vi "CST handler.vi"(0 "System no.":i32=1 min=1 max=4 step=1, 2 "Axis ID's In":string[](array[string]), 3 "Stage names In":string[](array[string]), 5 "error in":errorcluster, 6 "Query SAI? ALL?":bool=TRUE, 7 "Dialog?":bool=TRUE caption="Use dialog to define\nconnected stages?") -> (16 "Axis ID's Out":string[](array[string]), 17 "Stage names Out":string[](array[string]), 19 "error out":errorcluster)   [LabVIEW 2026]
doc: "Defines connected stages for axes, depending on several selections. Requires SAI.vi, SAI?.vi, CST?.vi and ERR?.vi. For Query SAI? ALL? = TRUE, VI determines connected axes by querying SAI? ALL. For Query SAI? = FALSE; Axis ID's IN must contain the correct identifiers of all connected axes. Use dialog to define connected stages? determines if a dialog pops up for the stage selection. If this control is set to FALSE, Stage names In must contain the correct stage names for all connected axes. Empty fields are substituted with \"NOSTAGE\". \n\nC-877, C-884, C-891: Command is available via USB interface only.\nC-867, E-871, E-873: Command is available via USB, USB DaisyChain or RS232 DaisyChain interface only.\nPollux: See HydraPollux_GCS_DLL manual for specialities of the Pollux controller family regarding stage name settings."
panel:
  # "Defines connected stages for axes, depending on several selections. Requires SAI.vi, SAI?.vi, CST?.vi and ERR?.vi."
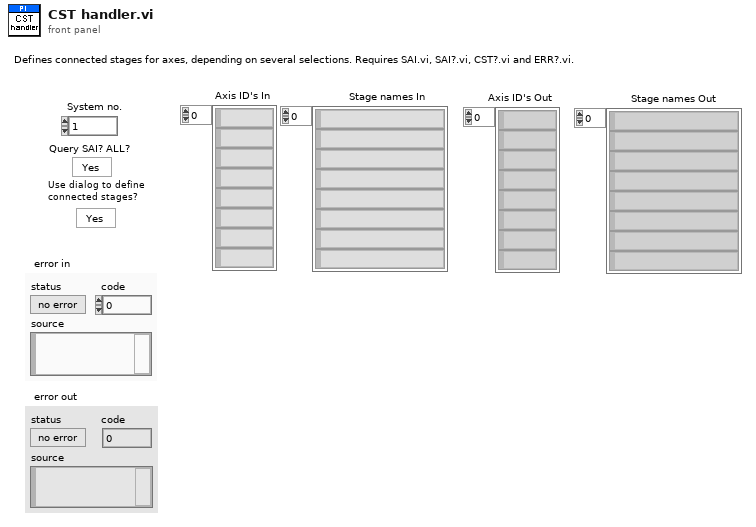
[diagram p1: front panel]
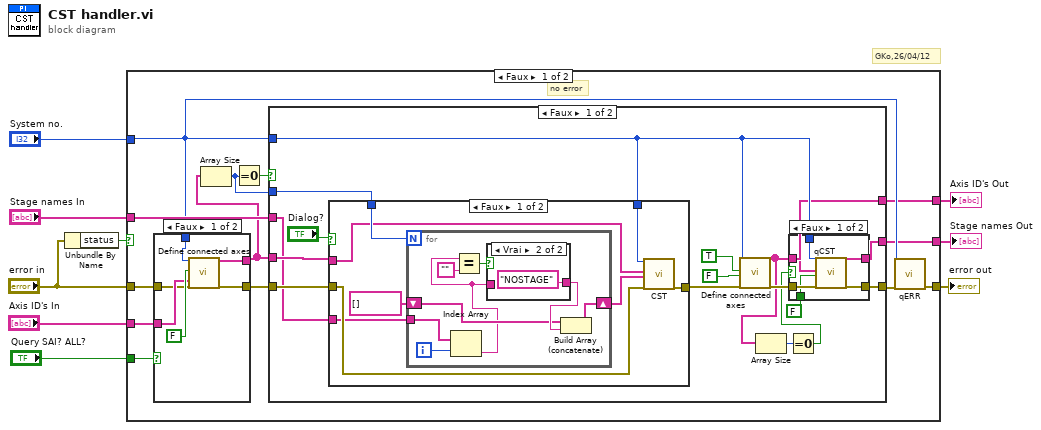
[diagram p0: block diagram]
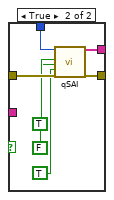
[diagram p2: hidden frame]
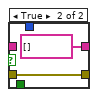
[diagram p3: hidden frame]
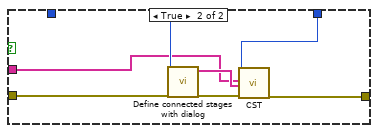
[diagram p5: hidden frame]
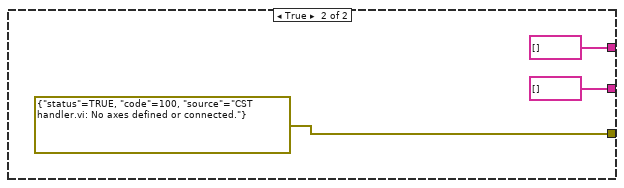
[diagram p6: hidden frame]
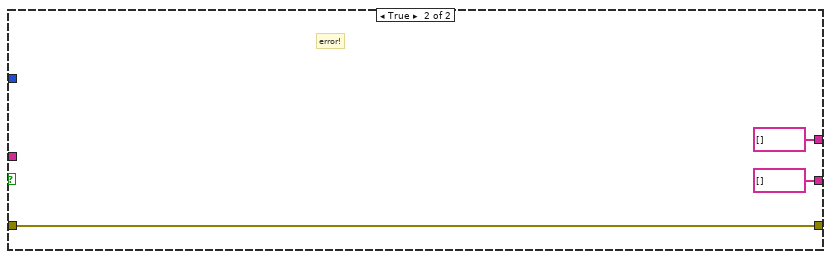
[diagram p7: hidden frame]
diagram:
  # "GKo,26/04/12"
  n1 = Unbundle By Name("error in") -> ("status"=w9:bool)
  n2 = case shown="Faux" w9 {
    tunnel: "error in" -> [w21 w89]
    tunnel: [w14 w89] -> w8
    tunnel: "Stage names In" -> [w22 _]
    tunnel: "System no." -> [w12 _]
    tunnel: "Query SAI? ALL?" -> [w19 _]
    tunnel: "Axis ID's In" -> [w18 _]
    tunnel: [w11 string[] [] ("Stage names")] -> w2
    tunnel: [w10 string[] [] ("Conn. Axes out")] -> w1
    frame False {
      # "no error"
      n3 = case shown="Faux" w19 {
        tunnel: w12 -> [w28 w35]
        tunnel: w21 -> [w25 w34]
        tunnel: [w23 w33] -> w20
        tunnel: [w24 w29] -> w16
        tunnel: w18 -> [w26 _]
        frame False {
          n4 = call "Define connected axes.vi"("System no."=w28, "Read from\ncontroller?"=FALSE ("Read from\ncontroller?"), "Conn. axes"=w26, "error in"=w25) -> ("Conn. Axes out"=w24:string[], "error out"=w23:errorcluster)  [unwired: 1 in, 13 out]
        }
        frame True {
          n5 = call "qSAI.vi"("System no."=w35, "Write to Global2?"=TRUE, "Invert order?"=FALSE, "SAI? ALL"=TRUE, "error in"=w34) -> ("Conn. axes"=w29:string[], "error out"=w33:errorcluster)  [unwired: 13 out]
        }
      }
      n6 = Array Size(array=w16) -> (size(s)=w15:i32)
      n7 = Equal To 0?(x=w15) -> (x = 0?=w17:bool)
      n8 = case shown="Faux" w17 {
        tunnel: [w42 errorcluster {"status"=TRUE, "code"=100, "source"="CST handler.vi: No axes defined or connected."} ("error out")] -> w13
        tunnel: w22 -> [w47 _]
        tunnel: w20 -> [w51 _]
        tunnel: w16 -> [w50 _]
        tunnel: w15 -> [w48 _]
        tunnel: w12 -> [w41 _]
        tunnel: [w40 string[] [] ("Stage names")] -> w11
        tunnel: [w38 string[] [] ("Conn. Axes out")] -> w10
        frame False {
          n9 = case shown="Faux" "Dialog?" {
            tunnel: w51 -> [w65 w81]
            tunnel: w41 -> [w64 w80]
            tunnel: w50 -> [w60 w79]
            tunnel: [w66 w78] -> w44
            tunnel: w48 -> [w67 _]
            tunnel: w47 -> [w63 _]
            frame False {
              n10 = for {
                N: w67 -> [_]
                shift-right: [w73] -> w61
                shift-left: string[] [] -> [w71]
                tunnel: w63 -> [w69]
                i -> [w70]
                n11 = Index Array(array=w69, index=w70) -> (element=w68:string)
                n12 = Equal?(x=w68, y="") -> (x = y?=w74:bool)
                n13 = case shown="Vrai" w74 {
                  tunnel: w68 -> [w76 _]
                  tunnel: [w76 "NOSTAGE" ("Stage names input")] -> w72
                  frame False {
                  }
                  frame True {
                  }
                }
                n14 = Build Array (concatenate)(w71, w72) -> (w73:string[])
              }
              n15 = call "CST.vi"("System no."=w64, "Axis ID's"=w60, "Stage names"=w61, "error in"=w65) -> ("error out"=w66:errorcluster)  [unwired: 15 out]
            }
            frame True {
              n16 = call "Define connected stages with dialog.vi"("System no."=w80, "error in"=w81) -> ("Stage selection"=w82:string[], "error out"=w83:errorcluster)  [unwired: 16 out]
              n17 = call "CST.vi"("System no."=w80, "Axis ID's"=w79, "Stage names"=w82, "error in"=w83) -> ("error out"=w78:errorcluster)  [unwired: 15 out]
            }
          }
          n18 = call "Define connected axes.vi"("System no."=w41, "Read from\ncontroller?"=TRUE ("Read from\nController"), "Invert\norder?"=FALSE ("Invert\nOrder"), "error in"=w44) -> ("Conn. Axes out"=w38:string[], "error out"=w43:errorcluster)  [unwired: 1 in, 13 out]
          n19 = Array Size(array=w38) -> (size(s)=w37:i32)
          n20 = Equal To 0?(x=w37) -> (x = 0?=w36:bool)
          n21 = case shown="Faux" w36 {
            tunnel: w43 -> [w57 w58]
            tunnel: [w56 w58] -> w42
            tunnel: w41 -> [w55 _]
            tunnel: [w54 string[] [] ("Stage names")] -> w40
            tunnel: FALSE ("All Axes?") -> [w53 _]
            tunnel: w38 -> [w52 _]
            frame False {
              n22 = call "qCST.vi"("System no."=w55, "Axes to query"=w52, "All Axes?"=w53, "error in"=w57) -> ("Stage names"=w54:string[], "error out"=w56:errorcluster)  [unwired: 1 in, 13 out]
            }
            frame True {
            }
          }
        }
        frame True {
        }
      }
      n23 = call "qERR.vi"("System no."=w12, "error in"=w13) -> ("error out"=w14:errorcluster)  [unwired: 17 out]
    }
    frame True {
      # "error!"
    }
  }
  "error out" <- w8
  "Axis ID's Out" <- w1
  "Stage names Out" <- w2
